vi "del img.vi"(8 "error in (no error)":errorcluster, 10 "id":i32, 11 "Test in":refnum<class "Test.lvclass">) -> (0 "error out":errorcluster, 3 "Test out":refnum<class "Test.lvclass">)   [LabVIEW 2013, in "DatenKlassen.lvlib" / "Test.lvclass"]
uses:
  Test.lvclass
  Image/img.lvclass
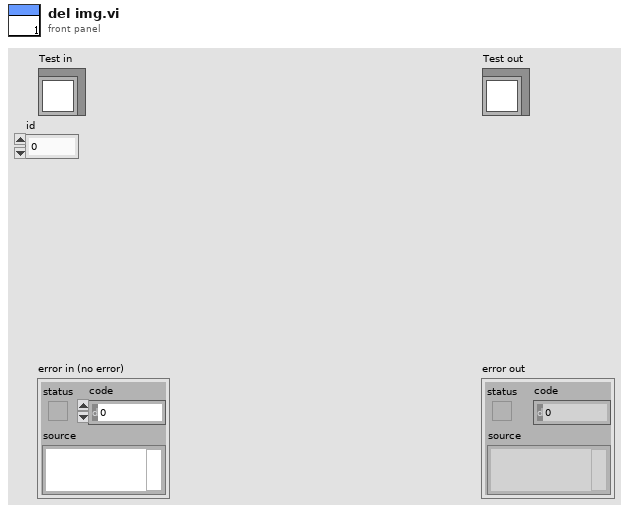
[diagram p1: front panel]
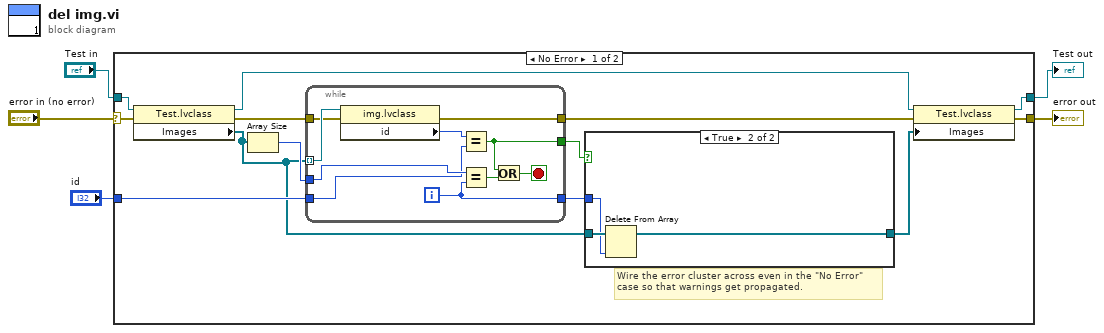
[diagram p0: block diagram]
diagram:
  n1 = case shown="No Error" "error in (no error)" {
    selector: "error in (no error)" -> [w9 w34]
    tunnel: [w6 w34] -> w4
    tunnel: [w10 w33] -> w2
    tunnel: "Test in" -> [w18 w33]
    tunnel: "id" -> [w15 _]
    frame No Error {
      # "Wire the error cluster across even in the \"No Error\"\ncase so that warnings get propagated."
      n2 = property class="Test.lvclass"(reference=w18, error in=w9) -> (reference out=w17:refnum<class "Test.lvclass">, error out=w8:errorcluster, "Images"=w13:refnum<class "img.lvclass">[])
      n3 = Array Size(array=w13) -> (size(s)=w16:i32)
      n4 = while {
        tunnel: w13 -> [w29] mode=indexing
        tunnel: w16 -> [w30]
        tunnel: w15 -> [w27]
        tunnel: [w26] -> w14
        tunnel: [w25] -> w12
        tunnel: w8 -> [w24]
        tunnel: [w23] -> w7
        i -> [w25]
        stop <- w32 stop-if-true
        n5 = property class="img.lvclass"(reference=w29, error in=w24) -> (error out=w23:errorcluster, "id"=w28:i32)  [unwired: 1 out]
        n6 = Equal?(x=w28, y=w27) -> (x = y?=w26:bool)
        n7 = Equal?(x=w30, y=w25) -> (x = y?=w31:bool)
        n8 = Or(x=w26, y=w31) -> (x .or. y?=w32:bool)
      }
      n9 = case shown="True" w14 {
        tunnel: w13 -> [w19 w22]
        tunnel: w12 -> [_ w21]
        tunnel: [w19 w20] -> w11
        frame False {
        }
        frame True {
          n10 = Delete From Array(array=w22, index=w21) -> (array with subset deleted=w20:refnum<class "img.lvclass">[])  [unwired: 1 in, 1 out]
        }
      }
      n11 = property class="Test.lvclass"(reference=w17, error in=w7, "Images"=w11) -> (reference out=w10:refnum<class "Test.lvclass">, error out=w6:errorcluster)
    }
    frame Error {
    }
  }
  "error out" <- w4
  "Test out" <- w2
